vi "Climber Arm Contol.vi"(10 "MotorControlDevRef":T1={"DeviceStatus"={"status"=FALSE, "code"=0, "source"=""}, "Type"=enum."PWM", "PWM"={"Digital Module"=enum."Digital Module 1", "PWM Channel"=enum."Invalid", "DeadBand"={"Name"="", "maxPositivePwm"=0, "minPositivePwm"=0, "centerPwm"=0, "maxNegativePwm"=0, "minNegativePwm"=0, "angularRange"=0}}, "CAN"={"Device Number"=0, "Control Mode"=enum."Percent VBus", "Semaphore"=refnum, "Max Vout"=12.0}, "Invert"=FALSE, "TransformRef"=refnum, "InvTransformRef"=refnum}) -> ()   [LabVIEW 2012]
uses:
  <vilib>/Rock Robotics/WPI/MotorControl/WPI_MotorControlDeviceRef.ctl
  <vilib>/Rock Robotics/SystemInterfaces/Typedef/FPGA_TypedefDigitalModule.ctl
  <vilib>/Rock Robotics/SystemInterfaces/DIO/FPGA_DIOPWMChannel.ctl
  <vilib>/Rock Robotics/WPI/PWM/WPI_PWMDeadband.ctl
  <vilib>/Rock Robotics/WPI/CAN/Jaguar/SubVIs/WPI_CANJaguar_ControlMode.ctl
  <vilib>/Rock Robotics/WPI/PWM/WPI_PWMTransform_ConPane.ctl
  Robot Global Data.vi
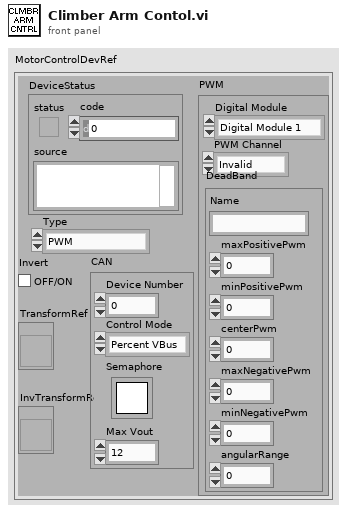
[diagram p1: front panel]
types:
  T1 = typedef "WPI_MotorControlDeviceRef.ctl" = cluster{"DeviceStatus":errorcluster, "Type":enum16{"PWM", "CAN"}, "PWM":cluster{"Digital Module":T2, "PWM Channel":T3, "DeadBand":T4}, "CAN":cluster{"Device Number":u8, "Control Mode":T5, "Semaphore":T6, "Max Vout":dbl}, "Invert":bool, "TransformRef":T7, "InvTransformRef":T7}
  T2 = typedef "FPGA_TypedefDigitalModule.ctl" = enum16{"Digital Module 1", "Digital Module 2"}
  T3 = typedef "FPGA_DIOPWMChannel.ctl" = enum8{"PWM 1", "PWM 2", "PWM 3", "PWM 4", "PWM 5", "PWM 6", "PWM 7", "PWM 8", "PWM 9", "PWM 10", "Invalid"}
  T4 = typedef "WPI_PWMDeadband.ctl" = cluster{"Name":string, "maxPositivePwm":i32, "minPositivePwm":i32, "centerPwm":i32, "maxNegativePwm":i32, "minNegativePwm":i32, "angularRange":u16}
  T5 = typedef "WPI_CANJaguar_ControlMode.ctl" = enum8{"Percent VBus", "Current", "Speed", "Position", "Voltage"}
  T6 = typedef "Semaphore RefNum" = refnum<k1>
  T7 = typedef "WPI_PWMTransform_ConPane.ctl" = refnum<vi>
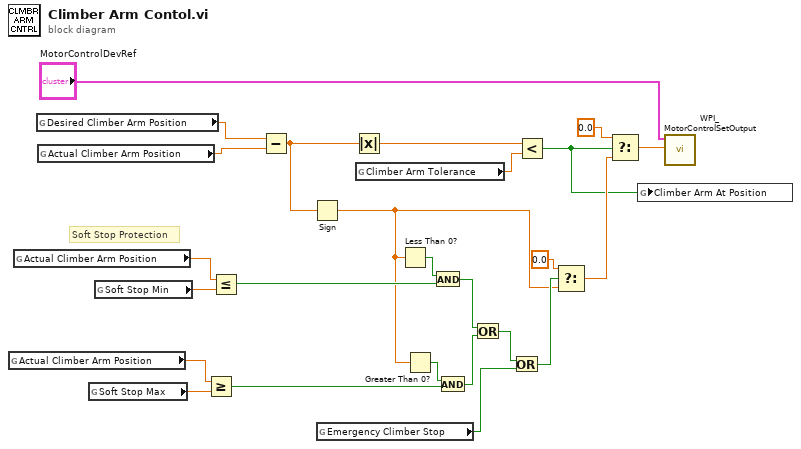
[diagram p0: block diagram]
diagram:
  # "Soft Stop Protection"
  n1 = global read "Robot Global Data.vi" "Actual Climber Arm Position"() -> (w12:dbl)
  n2 = global read "Robot Global Data.vi" "Actual Climber Arm Position"() -> (w18:dbl)
  n3 = global read "Robot Global Data.vi" "Desired Climber Arm Position"() -> (w24:dbl)
  n4 = global read "Robot Global Data.vi" "Actual Climber Arm Position"() -> (w23:dbl)
  n5 = global read "Robot Global Data.vi" "Soft Stop Max"() -> (w13:dbl)
  n6 = global read "Robot Global Data.vi" "Soft Stop Min"() -> (w19:dbl)
  n7 = Greater Or Equal?(x=w12, y=w13) -> (x >= y?=w10:bool)
  n8 = Less Or Equal?(x=w18, y=w19) -> (x <= y?=w17:bool)
  n9 = Subtract(x=w24, y=w23) -> (x-y=w4:dbl)
  n10 = Sign(1:w4) -> (0:w1:dbl)
  n11 = global read "Robot Global Data.vi" "Emergency Climber Stop"() -> (w6:bool)
  n12 = Absolute Value(x=w4) -> (abs(x)=w25:dbl)
  n13 = global read "Robot Global Data.vi" "Climber Arm Tolerance"() -> (w20:dbl)
  n14 = Less Than 0?(x=w1) -> (x < 0?=w16:bool)
  n15 = Greater Than 0?(x=w1) -> (x > 0?=w11:bool)
  n16 = And(x=w16, y=w17) -> (x .and. y?=w9:bool)
  n17 = And(x=w11, y=w10) -> (x .and. y?=w8:bool)
  n18 = Or(x=w9, y=w8) -> (x .or. y?=w7:bool)
  n19 = Or(x=w7, y=w6) -> (x .or. y?=w5:bool)
  n20 = Less?(x=w25, y=w20) -> (x < y?=w3:bool)
  n21 = Select(t=0.0, s=w5, f=w1) -> (s? t:f=w14:dbl)
  n22 = Select(t=0.0, s=w3, f=w14) -> (s? t:f=w21:dbl)
  n23 = global write "Robot Global Data.vi" "Climber Arm At Position"(w3) -> ()
  n24 = call <vilib>:"WPI_MotorControlSetOutput.vi"("Output"=w21, "MotorControlDevRef"="MotorControlDevRef") -> ()  [unwired: 7 in, 3 out]
